vi "main1.vi"() -> ()   [LabVIEW 2009]
uses:
  <vilib>/Instr/_visa.llb/VISA Configure Serial Port (Instr).vi
panel:
  in  "停止":bool
  in  "delay before read (ms)":u32=500 caption="读取前延时(ms)"
  in  "flow control":u16(ring) caption="流程控制" items=["无"=0, "XON/XOFF"=1, "RTS/CTS"=2, "DTR/DSR"=4]
  in  "stop bits":u16(ring)=10 caption="停止位" items=["1.0"=10, "1.5"=15, "2.0"=20]
  in  "parity":u16(ring) caption="奇偶" items=["无", "奇", "偶", "标记", "空格"]
  in  "data bits":u16=8 caption="数据比特" min=5 max=8 step=1
  in  "read":bool=TRUE caption="读取"
  in  "write":bool=TRUE caption="写入"
  out "bytes read":u32 caption="读取的字节"
  out "read string":string caption="读取字符串"
  in  "VISA resource name":refnum<visa-resource-name>="COM1" caption="VISA资源名称"
  in  "baud rate":u32=9600 caption="波特率"
  in  "Spoken Text":string
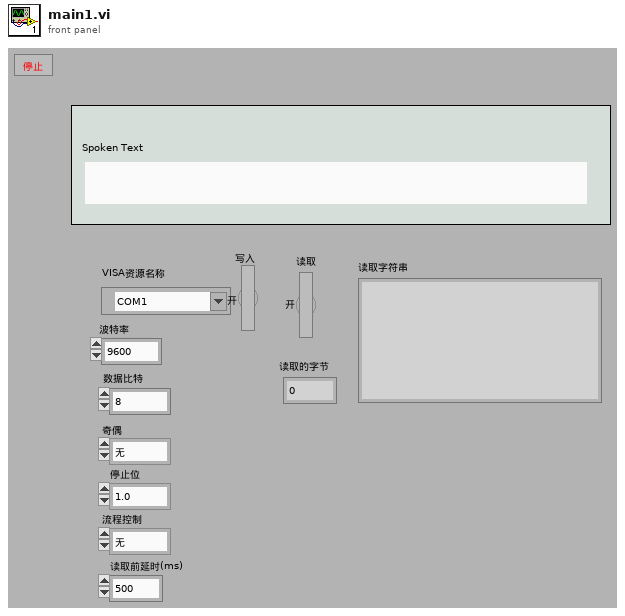
[diagram p1: front panel]
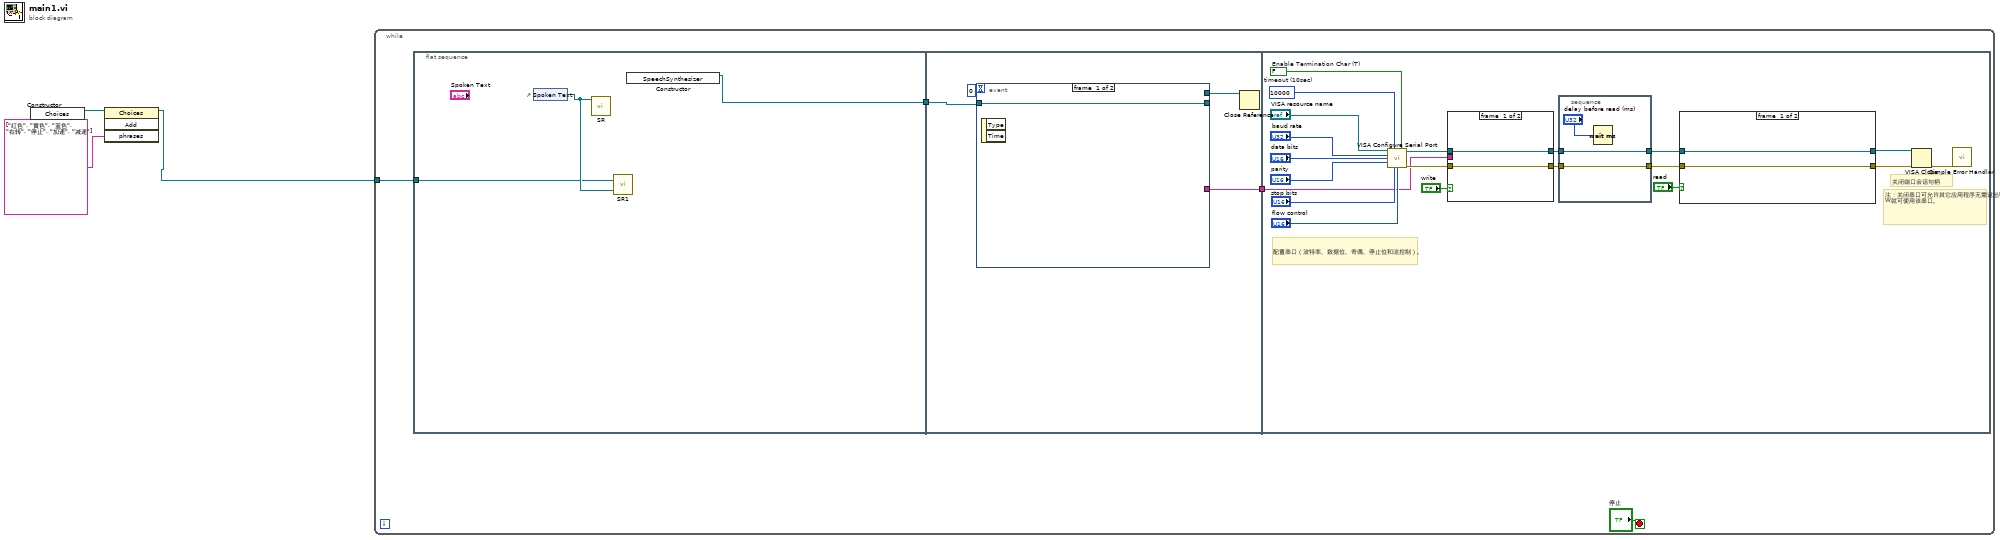
[diagram p0: block diagram]
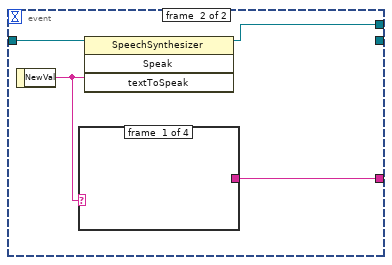
[diagram p2: hidden frame]
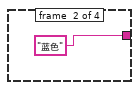
[diagram p3: hidden frame]
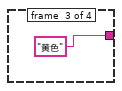
[diagram p4: hidden frame]
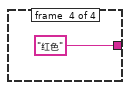
[diagram p5: hidden frame]
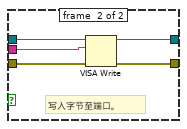
[diagram p6: hidden frame]
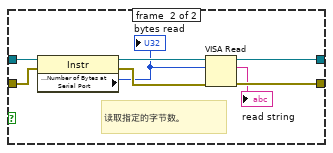
[diagram p7: hidden frame]
diagram:
  n1 = constructor class="Choices"() -> (reference out=w2:refnum<k24>)  [unwired: 3 in, 2 out]
  n2 = invoke class="Choices" method="Add"(reference=w2, "phrases"=string[] ["红色", "黄色", "蓝色", "右转", "停止", "加速", "减速"]) -> (reference out=w1:refnum<k24>)  [unwired: 2 in, 3 out]
  n3 = while {
    tunnel: w1 -> [w5]
    stop <- "停止" stop-if-true
    n4 = flat-sequence {
      tunnel: [w10] -> w7
      tunnel: w5 -> [w8]
      tunnel: w7 -> [w14]
      tunnel: [w12] -> w6
      tunnel: w6 -> [w23]
      frame #0 {
        n5 = control-ref of="Spoken Text"() -> (w9:refnum<vi>)
        n6 = call "SR.vi"("Spoken text box"=w9) -> ()  [unwired: 6 in, 1 out]
        n7 = call "SR1.vi"("Spoken text box"=w9, "new reference"=w8) -> ()  [unwired: 1 out]
        n8 = constructor class="SpeechSynthesizer"() -> (reference out=w10:refnum<k24>)  [unwired: 3 in, 2 out]
      }
      frame #1 {
        n9 = event shown="[1] \"Spoken Text\": 值改变" {
          selector: _ -> [_ _]
          dyn-events: _ -> [_ _]
          timeout: 0 -> [_ _]
          tunnel: w14 -> [w15 w19]
          tunnel: [w15 _] -> _
          tunnel: [_ w17] -> w13
          tunnel: [_ w16] -> w12
          event #0 {
            n10 = event-data() -> ()  [unwired: 1 in, 2 out]
          }
          event #1 {
            n11 = event-data() -> ("NewVal"=w18:string)  [unwired: 1 in]
            n12 = case shown="\"红色\"" w18 {
              tunnel: [_ "蓝色" "黄色" "红色"] -> w16
              frame #0 {
              }
              frame #1 {
              }
              frame #2 {
              }
              frame #3 {
              }
            }
            n13 = invoke class="SpeechSynthesizer" method="Speak"(reference=w19, "textToSpeak"=w18) -> (reference out=w17:refnum<k24>)  [unwired: 2 in, 3 out]
          }
        }
        n14 = Close Reference(reference=w13) -> ()  [unwired: 1 in, 1 out]
      }
      frame #2 {
        w32 = FALSE  # Enable Termination Char (T)
        w33 = u32 10000  # timeout (10sec)
        # "注：关闭串口可允许其它应用程序无需退出LabVIEW就可使用该串口。"
        # "配置串口（波特率、数据位、奇偶、停止位和流控制）。"
        # "关闭端口会话句柄"
        n15 = call-poly "VISA Configure Serial Port"("VISA resource name"="VISA resource name", "timeout (10sec)"=w33, "Enable Termination\nChar (T)"=w32, "baud rate (9600)"="baud rate", "data bits (8)"="data bits", "parity (0:none)"="parity", "stop bits (10: 1 bit)"="stop bits", "flow control (0:none)"="flow control") -> ("VISA resource name out"=w38:refnum<visa-resource-name>, "error out"=w39:errorcluster)  [unwired: 1 in, 5 out]
        n16 = case shown="真" "write" {
          tunnel: [w47 w52] -> w27
          tunnel: w38 -> [w46 w51]
          tunnel: w39 -> [w47 w50]
          tunnel: [w46 w49] -> w25
          tunnel: w23 -> [_ w48]
          frame #0 {
          }
          frame #1 {
            # "写入字节至端口。"
            n17 = VISA Write(VISA resource name=w51, write buffer=w48, error in (no error)=w50) -> (VISA resource name out=w49:refnum<visa-resource-name>, error out=w52:errorcluster)  [unwired: 1 out]
          }
        }
        n18 = stacked-sequence {
          tunnel: w27 -> [w45]
          tunnel: [w45] -> w26
          tunnel: w25 -> [w44]
          tunnel: [w44] -> w24
          frame #0 {
            n19 = Wait (ms)(milliseconds to wait="delay before read (ms)") -> ()  [unwired: 1 out]
          }
        }
        n20 = case shown="真" "read" {
          tunnel: w26 -> [w54 w58]
          tunnel: [w54 w62] -> w37
          tunnel: [w53 w61] -> w36
          tunnel: w24 -> [w53 w60]
          frame #0 {
          }
          frame #1 {
            # "读取指定的字节数。"
            n21 = property class="Instr"(reference=w60, error in=w58) -> (reference out=w59:refnum<visa-resource-name>, error out=w57:errorcluster, "Serial Settings:Number of Bytes at Serial Port"=w55:u32)
            "bytes read" <- w55
            n22 = VISA Read(VISA resource name=w59, byte count=w55, error in (no error)=w57) -> (VISA resource name out=w61:refnum<visa-resource-name>, read buffer=→"read string":string, error out=w62:errorcluster)  [unwired: 1 out]
          }
        }
        n23 = VISA Close(VISA resource name=w36, error in (no error)=w37) -> (error out=w35:errorcluster)
        n24 = call <vilib>:"Simple Error Handler.vi"("error in (no error)"=w35) -> ()  [unwired: 1 in, 8 out]
      }
    }
  }
